vi "Rendezvous.vi"() -> ()   [LabVIEW 2019]
uses:
  <vilib>/measure/NI_MABase.lvlib
panel:
  out "String":string
  out "LED-3":bool
  out "LED-2":bool
  out "LED-1":bool
  out "L-3: 1s":waveform(dbl)(graph)={"t0"=timestamp(206.0 s since 1904-01-01), "dt"=0.001, "Y"=array[1000 elements]} caption="L-2"
  out "L-2: 4s":waveform(dbl)(graph)={"t0"=timestamp(206.0 s since 1904-01-01), "dt"=0.001, "Y"=array[1000 elements]} caption="L-2"
  out "L-1: 2s":waveform(dbl)(graph)={"t0"=timestamp(86.0 s since 1904-01-01), "dt"=0.001, "Y"=array[1000 elements]}
  in  "?":bool
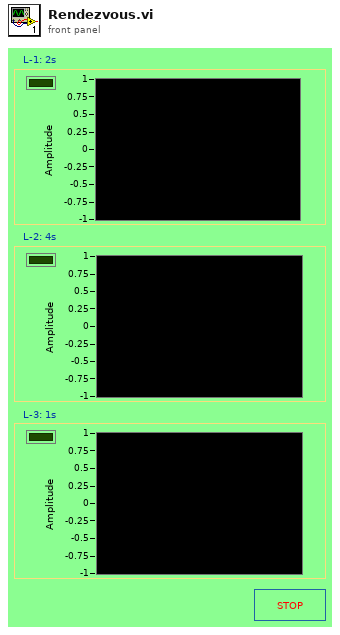
[diagram p1: front panel]
types:
  T1 = typedef "Rendezvous RefNum" = refnum<k1>
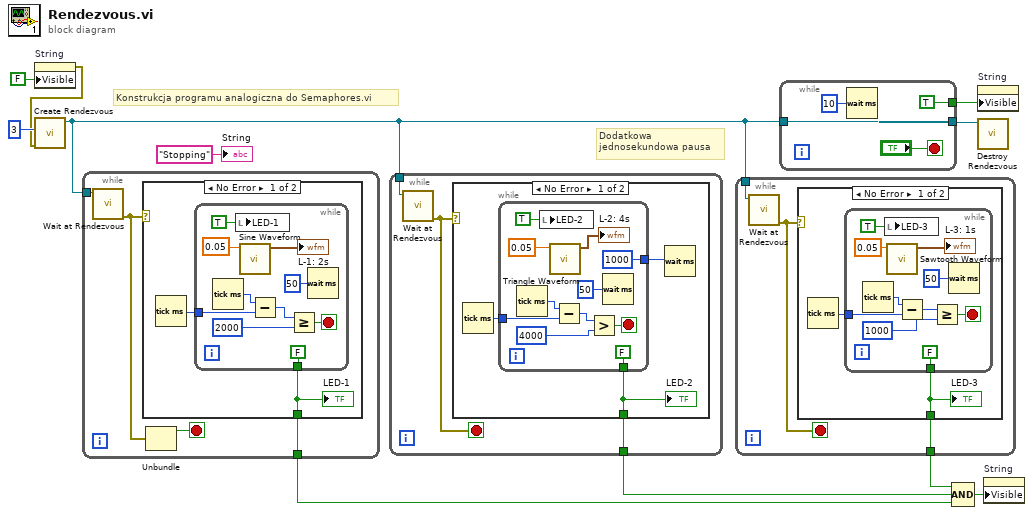
[diagram p0: block diagram]
diagram:
  # "Dodatkowa\njednosekundowa pausa"
  # "Konstrukcja programu analogiczna do Semaphores.vi"
  n1 = property on="String" class="Str"("Visible"=FALSE) -> (error out=w6:errorcluster)  [unwired: 2 in, 1 out]
  n2 = call <vilib>:"Create Rendezvous.vi"("error in (no error)"=w6, "size (2)"=3) -> ("rendezvous"=w9:T1)  [unwired: 3 in, 2 out]
  n3 = while {
    tunnel: w9 -> [w15]
    tunnel: [w13] -> w2
    stop <- w14 stop-if-true
    n4 = call <vilib>:"Wait at Rendezvous.vi"("rendezvous"=w15) -> ("error out"=w12:errorcluster)  [unwired: 4 in, 2 out]
    n5 = case shown="No Error" w12 {
      tunnel: [w16 _] -> w13
      frame No Error {
        n6 = Tick Count (ms)() -> (millisecond timer value=w17:u32)
        n7 = while {
          tunnel: w17 -> [w24]
          tunnel: [FALSE ("LED-1")] -> w16
          stop <- w22 stop-if-true
          n8 = Tick Count (ms)() -> (millisecond timer value=w25:u32)
          n9 = local write "LED-1"(TRUE ("LED-1")) -> ()
          n10 = call <vilib>:"Sine Waveform.vi"("frequency"=0.05) -> ("signal out"=→"L-1: 2s":waveform(dbl))  [unwired: 9 in, 1 out]
          n11 = Subtract(x=w25, y=w24) -> (x-y=w20:u32)
          n12 = Greater Or Equal?(x=w20, y=u32 2000) -> (x >= y?=w22:bool)
          n13 = Wait (ms)(milliseconds to wait=u32 50) -> ()  [unwired: 1 out]
        }
        "LED-1" <- w16
      }
      frame Error {
      }
    }
    n14 = Unbundle(w12) -> ("status"=w14:bool)  [unwired: 2 out]
  }
  n15 = while {
    tunnel: w9 -> [w30]
    tunnel: [w28] -> w3
    stop <- w29 stop-if-true
    n16 = call <vilib>:"Wait at Rendezvous.vi"("rendezvous"=w30) -> ("error out"=w29:errorcluster)  [unwired: 4 in, 2 out]
    n17 = case shown="No Error" w29 {
      tunnel: [w31 _] -> w28
      frame No Error {
        n18 = Tick Count (ms)() -> (millisecond timer value=w33:u32)
        n19 = while {
          tunnel: w33 -> [w41]
          tunnel: [u32 1000 ("x")] -> w32
          tunnel: [FALSE ("LED-2")] -> w31
          stop <- w39 stop-if-true
          n20 = Tick Count (ms)() -> (millisecond timer value=w42:u32)
          n21 = local write "LED-2"(TRUE ("LED-2")) -> ()
          n22 = call <vilib>:"Triangle Waveform.vi"("frequency"=0.05) -> ("signal out"=→"L-2: 4s":waveform(dbl))  [unwired: 9 in, 1 out]
          n23 = Subtract(x=w42, y=w41) -> (x-y=w37:u32)
          n24 = Greater?(x=w37, y=u32 4000) -> (0:w39:bool)
          n25 = Wait (ms)(milliseconds to wait=u32 50) -> ()  [unwired: 1 out]
        }
        "LED-2" <- w31
        n26 = Wait (ms)(milliseconds to wait=w32) -> ()  [unwired: 1 out]
      }
      frame Error {
      }
    }
  }
  n27 = while {
    tunnel: w9 -> [w47]
    tunnel: [w46] -> w4
    stop <- w45 stop-if-true
    n28 = call <vilib>:"Wait at Rendezvous.vi"("rendezvous"=w47) -> ("error out"=w45:errorcluster)  [unwired: 4 in, 2 out]
    n29 = case shown="No Error" w45 {
      tunnel: [w48 _] -> w46
      frame No Error {
        n30 = Tick Count (ms)() -> (millisecond timer value=w49:u32)
        n31 = while {
          tunnel: w49 -> [w56]
          tunnel: [FALSE ("LED-3")] -> w48
          stop <- w54 stop-if-true
          n32 = Tick Count (ms)() -> (millisecond timer value=w57:u32)
          n33 = local write "LED-3"(TRUE ("LED-3")) -> ()
          n34 = call <vilib>:"Sawtooth Waveform.vi"("frequency"=0.05) -> ("signal out"=→"L-3: 1s":waveform(dbl))  [unwired: 9 in, 1 out]
          n35 = Subtract(x=w57, y=w56) -> (x-y=w52:u32)
          n36 = Greater Or Equal?(x=w52, y=u32 1000) -> (x >= y?=w54:bool)
          n37 = Wait (ms)(milliseconds to wait=u32 50) -> ()  [unwired: 1 out]
        }
        "LED-3" <- w48
      }
      frame Error {
      }
    }
  }
  n38 = while {
    tunnel: w9 -> [w63]
    tunnel: [w63] -> w11
    tunnel: [TRUE] -> w5
    stop <- "?" stop-if-true
    n39 = Wait (ms)(milliseconds to wait=u32 10) -> ()  [unwired: 1 out]
  }
  n40 = Compound Arithmetic op=AND(w4, w3, w2) -> (w1:bool)
  n41 = property on="String" class="Str"("Visible"=w5) -> ()  [unwired: 2 in, 2 out]
  n42 = call <vilib>:"Destroy Rendezvous.vi"("rendezvous"=w11) -> ()  [unwired: 5 in, 2 out]
  n43 = property on="String" class="Str"("Visible"=w1) -> ()  [unwired: 2 in, 2 out]
  "String" <- "Stopping" ("String")
